vi "Actor Core.vi"(8 "error in":errorcluster, 11 "Controller in":refnum<class "Controller.lvclass">) -> (0 "error out":errorcluster, 3 "Actor out":refnum<class "Actor.lvclass">)   [LabVIEW 2026, in "Controller Actor.lvlib" / "Controller.lvclass"]
doc: "(<B>Filename</B>: Actor Framework.lvlib:Actor.lvclass:Actor Core.vi)\n\nReceives messages to the actor, reacts to them, and initiates any error handling that may shut the actor down.\n\nDescendant classes may override this VI to append parallel tasks for the actor to complete while it handles messages. Overrides use the Call Parent Method node."
uses:
  Controller.lvclass
  C:/Program Files/National Instruments/LabVIEW 2026/vi.lib/ActorFramework/Actor/Actor.lvclass
  <vilib>/ActorFramework/Actor/Actor.lvclass
  <vilib>/ActorFramework/Actor/Actor.lvclass/Actor.ctl
  <vilib>/ActorFramework/Message Enqueuer/Message Enqueuer.lvclass/Message Enqueuer.ctl
  Controller Messages/Update lookup table of devices on system Msg/Update lookup table of devices on system Msg.lvclass/Update lookup table of devices on system Msg.ctl
  <vilib>/ActorFramework/Message Enqueuer/Init from Existing Queue.vi
  <vilib>/ActorFramework/Message Enqueuer/Enqueue.vi
  Controller Messages/Update lookup table of devices on system Msg/Update lookup table of devices on system Msg.lvclass
  C:/Program Files/National Instruments/LabVIEW 2026/vi.lib/ActorFramework/Message/Message.lvclass
  <vilib>/ActorFramework/Message Priority Queue/Priority Enqueue.vi
  <vilib>/ActorFramework/Message Enqueuer/Message Enqueuer.lvclass
  Controller.lvclass/Controller.ctl
  C:/Users/E2013170/Documents/GitHub/Measurement-Utility-Reference/components/MAL-Framework/user.lib/Common Components/Controller/Controller.lvclass
panel:
  out "Resources out":refnum<k20>[](array[refnum])
  out "error out 2":errorcluster caption="error out"
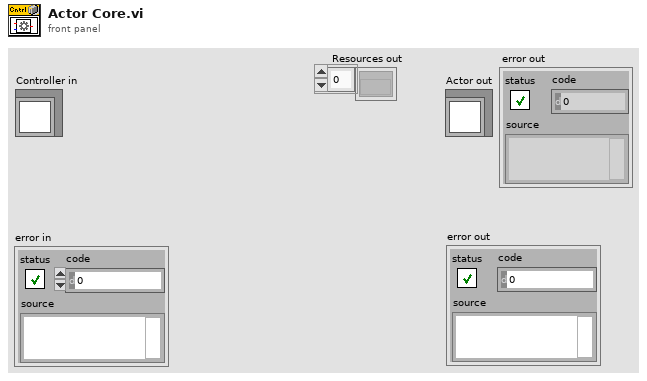
[diagram p1: front panel]
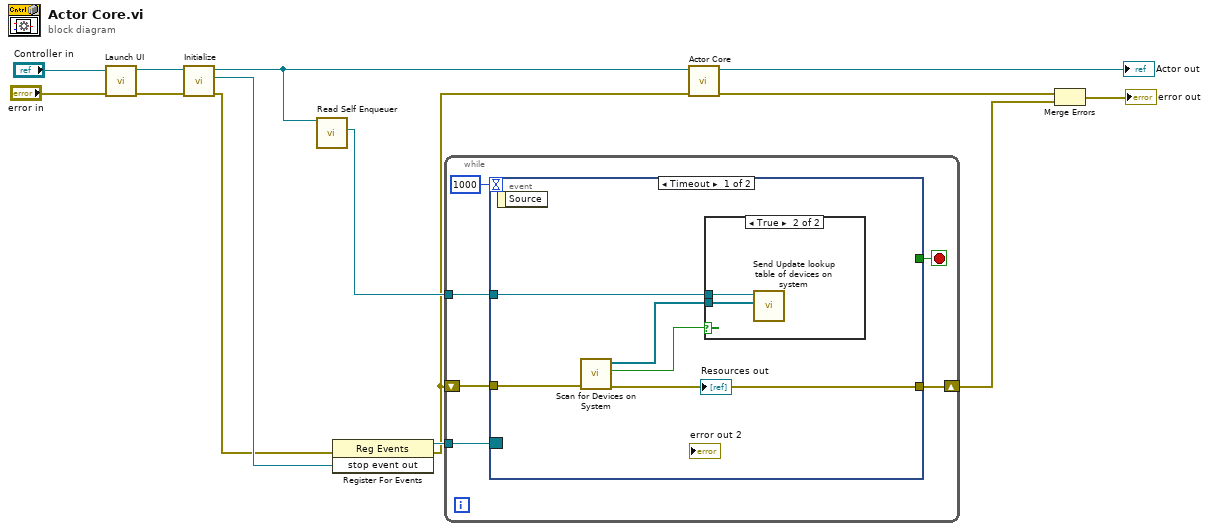
[diagram p0: block diagram]
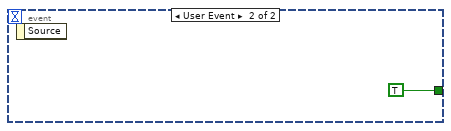
[diagram p3: hidden frame]
diagram:
  n1 = call-dynamic "Launch UI.vi"("error in (no error)"="error in", "Controller In"="Controller in") -> ("error out"=w9:errorcluster, "Controller Out"=w11:refnum<class "Controller.lvclass">)  [unwired: 8 in]
  n2 = call-dynamic "Initialize.vi"("error in (no error)"=w9, "Controller Actor.lvlib:Controller.lvclass"=w11) -> ("error out"=w2:errorcluster, "stop event out"=w7:refnum<user-event>, "Controller out"=w8:refnum<class "Controller.lvclass">)  [unwired: 7 in]
  n3 = call <vilib>:"Read Self Enqueuer.vi"("Actor"=w8) -> ("Self Enqueuer"=w6:refnum<class "Message Enqueuer.lvclass">)  [unwired: 10 in]
  n4 = register-events(error in=w2, w7) -> (reference out=w5:refnum<event-registration>, error out=w1:errorcluster)  [unwired: 1 in]
  n5 = while {
    tunnel: w6 -> [w20]
    tunnel: w5 -> [w19]
    shift-right: [w16] -> w3
    shift-left: w1 -> [w18]
    stop <- w17 stop-if-true
    n6 = event shown="[0] Timeout" {
      selector: w19 -> [_ _]
      dyn-events: _ -> [_ _]
      timeout: 1000 -> [_ _]
      tunnel: w20 -> [w25 _]
      tunnel: w18 -> [w24 _]
      tunnel: [_ TRUE] -> w17
      tunnel: [w22 _] -> w16
      event Timeout {
        n7 = event-data() -> ()  [unwired: 1 in, 1 out]
        n8 = call "Scan for Devices on System.vi"("error in (no error)"=w24) -> ("error out"=w22:errorcluster, "Changed?"=w21:bool, "Resources out"=w23:refnum<k20>[])  [unwired: 8 in]
        n9 = case shown="True" w21 {
          tunnel: w25 -> [_ w26]
          tunnel: w23 -> [_ w27]
          frame False {
          }
          frame True {
            n10 = call "Send Update lookup table of devices on system.vi"("Hardware Resources"=w27, "Message Enqueuer"=w26) -> ()  [unwired: 8 in, 2 out]
          }
        }
      }
      event User Event {
        n11 = event-data() -> ()  [unwired: 1 in, 1 out]
      }
    }
  }
  n12 = call-parent "Actor Core.vi"("error in"=w1, "Actor in"=w8) -> ("error out"=w14:errorcluster, "Actor out"=→"Actor out":refnum<class "Actor.lvclass">)  [unwired: 8 in]
  n13 = Merge Errors(w14, w3) -> (→"error out":errorcluster)
